vi "Inst_CNT90.vi"(8 "error in":errorcluster, 10 "All Message Queues in":T1, 11 "Prueba31 in":refnum<class "Prueba07.lvclass">) -> (0 "error out":errorcluster)   [LabVIEW 2019, in "Prueba07.lvclass"]
uses:
  Prueba07.lvclass
  QMH/Message Queue/All Message Queues.ctl
  QMH/Message Queue/Message Cluster.ctl
  Prueba07.lvclass/Prueba07.ctl
  <vilib>/Utility/error.llb/Error Cluster From Error Code.vi
  QMH/Message Queue/Enqueue Message (Single).vi
  <vilib>/ErrorRing/Error Ring.xnode
  QMH/Message Queue/Message Queue.lvlib
  Instrumento/CNT90/CNT90.lvclass
panel:
  out "All States":string[](array[string])
  out "Actual State":string
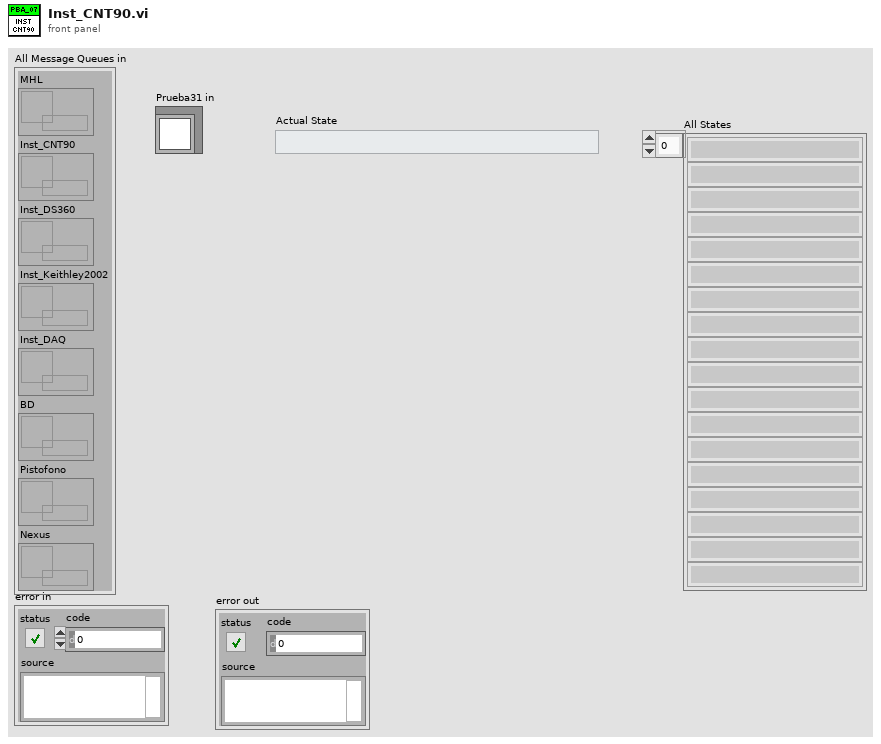
[diagram p1: front panel]
types:
  T1 = typedef "Message Queue.lvlib/All Message Queues.ctl" = cluster{"MHL":refnum<queue>, "Inst_CNT90":refnum<queue>, "Inst_DS360":refnum<queue>, "Inst_Keithley2002":refnum<queue>, "Inst_DAQ":refnum<queue>, "BD":refnum<queue>, "Pistofono":refnum<queue>, "Nexus":refnum<queue>}
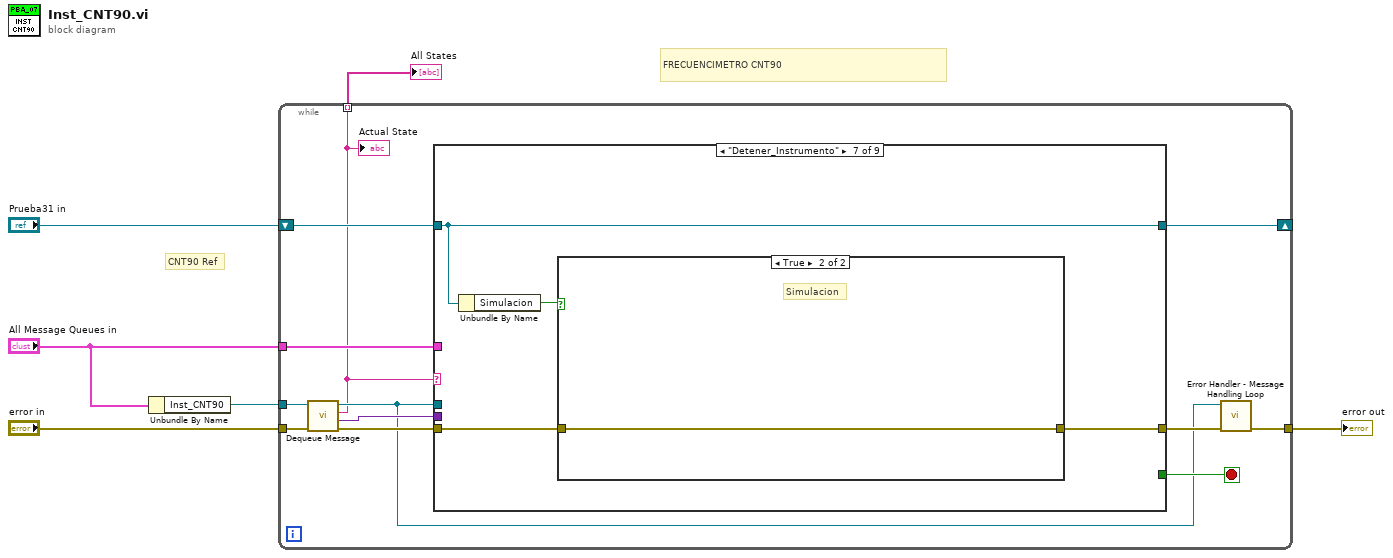
[diagram p0: block diagram]
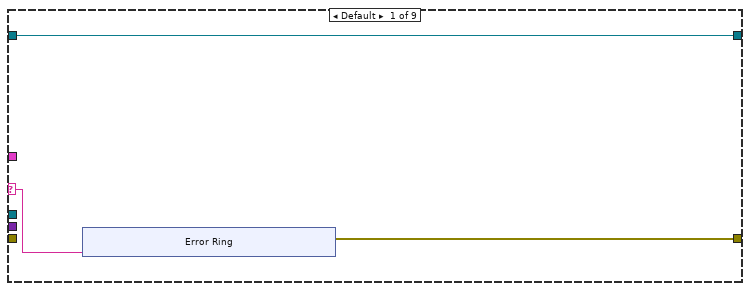
[diagram p2: hidden frame]
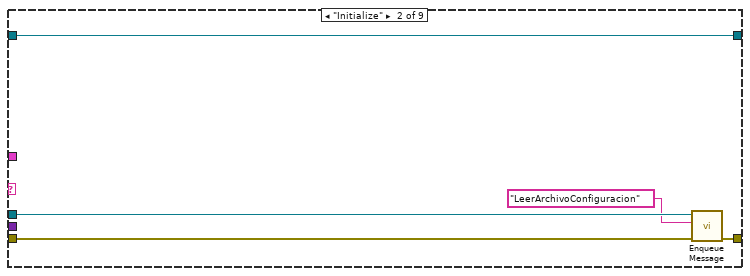
[diagram p3: hidden frame]
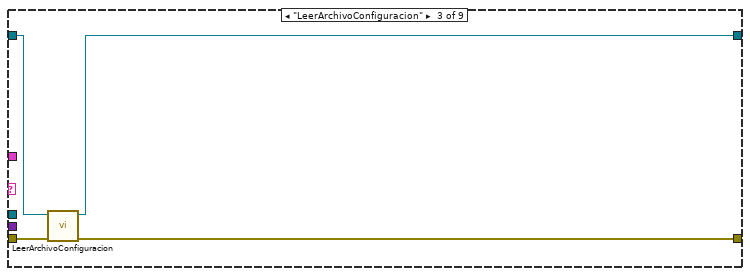
[diagram p4: hidden frame]
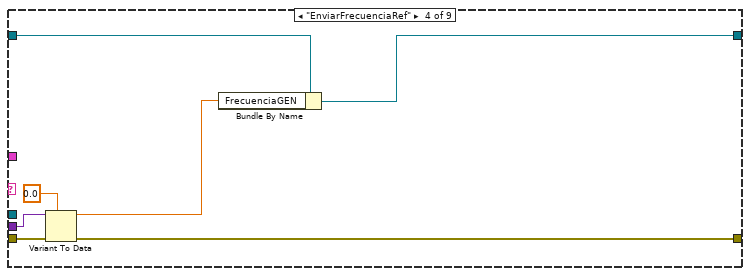
[diagram p5: hidden frame]
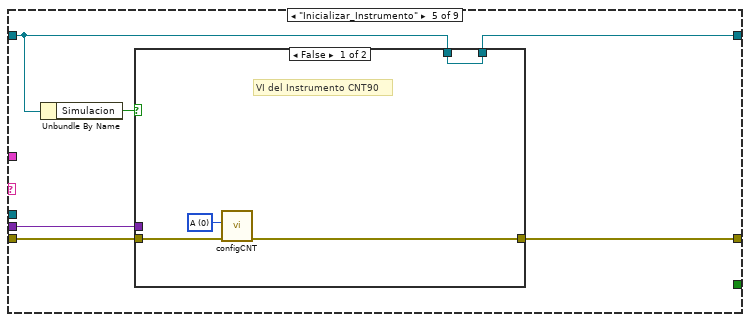
[diagram p6: hidden frame]
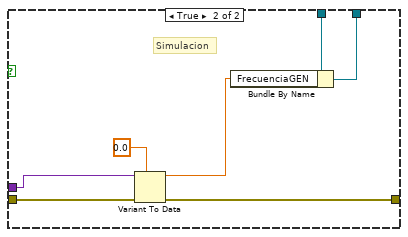
[diagram p7: hidden frame]
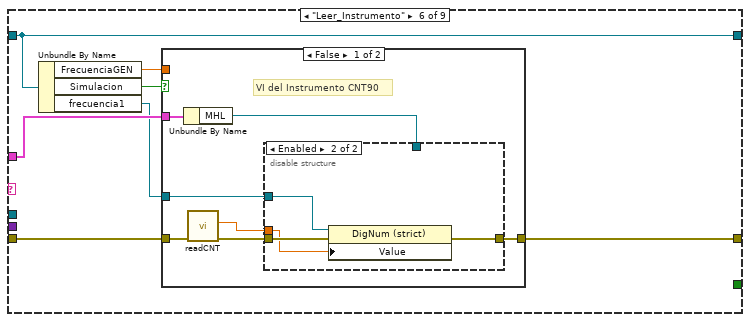
[diagram p8: hidden frame]
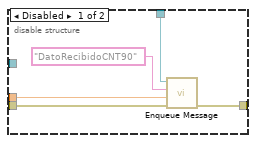
[diagram p9: hidden frame]
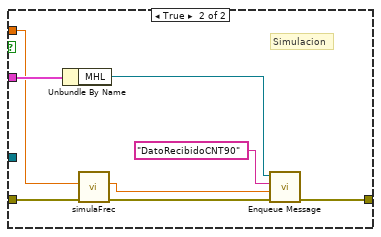
[diagram p10: hidden frame]
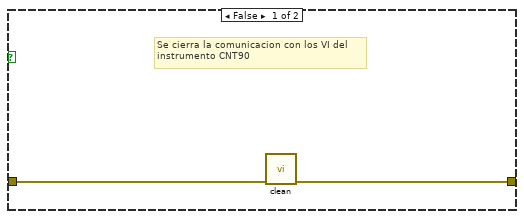
[diagram p11: hidden frame]
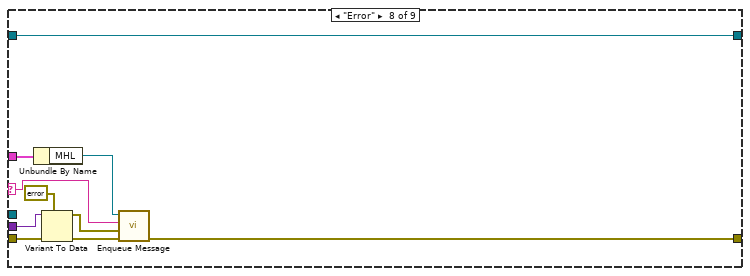
[diagram p12: hidden frame]
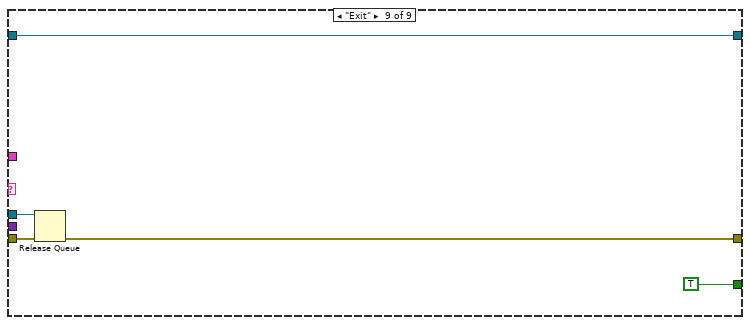
[diagram p13: hidden frame]
diagram:
  # "FRECUENCIMETRO CNT90"
  # "CNT90 Ref"
  n1 = Unbundle By Name("All Message Queues in") -> ("Inst_CNT90"=w4:refnum<queue>)
  n2 = while {
    tunnel: "error in" -> [w18]
    tunnel: w4 -> [w17]
    tunnel: "All Message Queues in" -> [w16]
    tunnel: [w9] -> w2
    shift-right: [w12] -> _
    shift-left: "Prueba31 in" -> [w15]
    tunnel: [w7] -> w1 mode=indexing
    stop <- w11 stop-if-true
    n3 = call "Dequeue Message.vi"("error in (no error)"=w18, "Message Queue"=w17) -> ("error out"=w13:errorcluster, "Message Data"=w14:variant, "Message"=w7:string, "dup Message Queue"=w8:refnum<queue>)  [unwired: 6 in]
    "Actual State" <- w7
    n4 = case shown="\"Detener_Instrumento\"" w7 {
      selector: w7 -> [w21 _ _ _ _ _ _ w104 _]
      tunnel: w16 -> [_ _ _ _ _ w64 _ w103 _]
      tunnel: w15 -> [w19 w33 w34 w39 w46 w66 w95 w101 w111]
      tunnel: w8 -> [_ w30 _ _ _ _ _ _ w113]
      tunnel: w14 -> [_ _ _ w42 w47 _ _ w107 _]
      tunnel: w13 -> [_ w31 w35 w43 w50 w68 w93 w108 w114]
      tunnel: [w20 w32 w37 w44 w48 w67 w96 w100 w110] -> w10
      tunnel: [w19 w33 w36 w40 w45 w66 w95 w101 w111] -> w12
      tunnel: [_ _ _ _ _ _ _ _ TRUE] -> w11
      frame Default {
        n5 = xnode "Error Ring"("parameter 0"=w21) -> ("error out"=w20:errorcluster)
      }
      frame "Initialize" {
        n6 = call-poly "Enqueue Message.vi"("error in (no error)"=w31, "Message"="LeerArchivoConfiguracion", "Message Queue"=w30) -> ("error out"=w32:errorcluster)  [unwired: 7 in, 1 out]
      }
      frame "LeerArchivoConfiguracion" {
        n7 = call "LeerArchivoConfiguracion.vi"("error in"=w35, "Prueba07 in"=w34) -> ("error out"=w37:errorcluster, "Prueba07 out"=w36:refnum<class "Prueba07.lvclass">)  [unwired: 8 in]
      }
      frame "EnviarFrecuenciaRef" {
        n8 = Variant To Data(error in=w43, type=0.0, Variant=w42) -> (data=w38:dbl, error out=w44:errorcluster)
        n9 = Bundle By Name(cluster=w39, "FrecuenciaGEN"=w38) -> (w40:refnum<class "Prueba07.lvclass">)
      }
      frame "Inicializar_Instrumento" {
        n10 = Unbundle By Name(w46) -> ("Simulacion"=w49:bool)
        n11 = case shown="False" w49 {
          tunnel: [w54 w60] -> w48
          tunnel: w50 -> [w53 w61]
          tunnel: w47 -> [_ w59]
          tunnel: w46 -> [w51 w57]
          tunnel: [w51 w56] -> w45
          frame False {
            w52 = 0 items=["A", "B"] ("Channel  1")
            # "VI del Instrumento CNT90"
            n12 = call "configCNT.vi"("error in (no error)"=w53, "Channel  1"=w52) -> ("error out"=w54:errorcluster)  [unwired: 8 in, 1 out]
          }
          frame True {
            # "Simulacion"
            n13 = Variant To Data(error in=w61, type=0.0, Variant=w59) -> (data=w55:dbl, error out=w60:errorcluster)
            n14 = Bundle By Name(cluster=w57, "FrecuenciaGEN"=w55) -> (w56:refnum<class "Prueba07.lvclass">)
          }
        }
      }
      frame "Leer_Instrumento" {
        n15 = Unbundle By Name(w66) -> ("FrecuenciaGEN"=w63:dbl, "Simulacion"=w65:bool, "frecuencia1"=w62:refnum<vi>)
        n16 = case shown="False" w65 {
          tunnel: [w72 w91] -> w67
          tunnel: w68 -> [w75 w88]
          tunnel: w64 -> [w71 w90]
          tunnel: w63 -> [_ w85]
          tunnel: w62 -> [w69 _]
          frame False {
            # "VI del Instrumento CNT90"
            n17 = Unbundle By Name(w71) -> ("MHL"=w70:refnum<queue>)
            n18 = call "readCNT.vi"("error in (no error)"=w75) -> ("error out"=w73:errorcluster, "medicion"=w74:dbl)  [unwired: 8 in, 1 out]
            n19 = disable-structure shown="Enabled" {
              disable-tunnel: w74 -> [w80 w81]
              disable-tunnel: w73 -> [w78 w84]
              disable-tunnel: [w77 w83] -> w72
              disable-tunnel: w70 -> [w76 _]
              disable-tunnel: w69 -> [_ w82]
              frame Disabled {
                n20 = call-poly "Enqueue Message.vi"("error in (no error)"=w78, "Message Data"=w80, "Message"="DatoRecibidoCNT90", "Message Queue"=w76) -> ("error out"=w77:errorcluster)  [unwired: 6 in, 1 out]
              }
              frame Enabled {
                n21 = property class="DigNum (strict)"(reference=w82, error in=w84, "Value"=w81) -> (error out=w83:errorcluster)  [unwired: 1 out]
              }
            }
          }
          frame True {
            # "Simulacion"
            n22 = Unbundle By Name(w90) -> ("MHL"=w89:refnum<queue>)
            n23 = call "simulaFrec.vi"("error in (no error)"=w88, "frec in"=w85) -> ("error out"=w87:errorcluster, "frec out"=w86:dbl)  [unwired: 7 in, 1 out]
            n24 = call-poly "Enqueue Message.vi"("error in (no error)"=w87, "Message Data"=w86, "Message"="DatoRecibidoCNT90", "Message Queue"=w89) -> ("error out"=w91:errorcluster)  [unwired: 6 in, 1 out]
          }
        }
      }
      frame "Detener_Instrumento" {
        n25 = Unbundle By Name(w95) -> ("Simulacion"=w94:bool)
        n26 = case shown="True" w94 {
          tunnel: [w98 w99] -> w96
          tunnel: w93 -> [w97 w99]
          frame False {
            # "Se cierra la comunicacion con los VI del\ninstrumento CNT90"
            n27 = call "clean.vi"("error in (no error)"=w97) -> ("error out"=w98:errorcluster)  [unwired: 9 in, 1 out]
          }
          frame True {
            # "Simulacion"
          }
        }
      }
      frame "Error" {
        n28 = Unbundle By Name(w103) -> ("MHL"=w102:refnum<queue>)
        n29 = Variant To Data(error in=w108, type=errorcluster {"status"=FALSE, "code"=0, "source"=""} ("error constant"), Variant=w107) -> (data=w105:errorcluster, error out=w106:errorcluster)
        n30 = call-poly "Enqueue Message.vi"("error in (no error)"=w106, "Message Data"=w105, "Message"=w104, "Message Queue"=w102) -> ("error out"=w100:errorcluster)  [unwired: 6 in, 1 out]
      }
      frame "Exit" {
        n31 = Release Queue(queue=w113, error in (no error)=w114) -> (error out=w110:errorcluster)  [unwired: 1 in, 2 out]
      }
    }
    n32 = call "Error Handler - Message Handling Loop.vi"("error in (no error)"=w10, "Message Queue"=w8) -> ("dup error in"=w9:errorcluster)  [unwired: 8 in, 1 out]
  }
  "error out" <- w2
  "All States" <- w1
